vi "FGV_PSP - IPS120 Status.vi"(4 "error in":errorcluster, 6 "Function":enum16{"write", "read"}(ring), 7 "Status":T1) -> (0 "error out":errorcluster, 3 "status":T1)   [LabVIEW 2016, in "IPS-120.lvlib" / "IPS-120-API.lvlib"]
uses:
  IPS-120-API.lvlib
  Typedefs/Status - Cluster.ctl
panel:
  # "Disabled calls to PSP 4/13/2018"
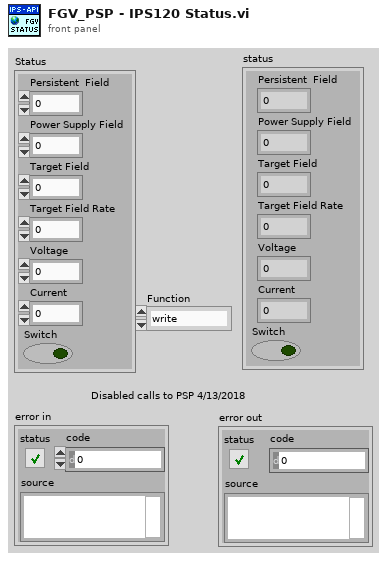
[diagram p1: front panel]
types:
  T1 = typedef "IPS-120.lvlib/IPS-120-API.lvlib/Status - Cluster.ctl" = cluster{"Persistent  Field":dbl, "Power Supply Field":dbl, "Target Field":dbl, "Target Field Rate":dbl, "Voltage":dbl, "Current":dbl, "Switch":bool}
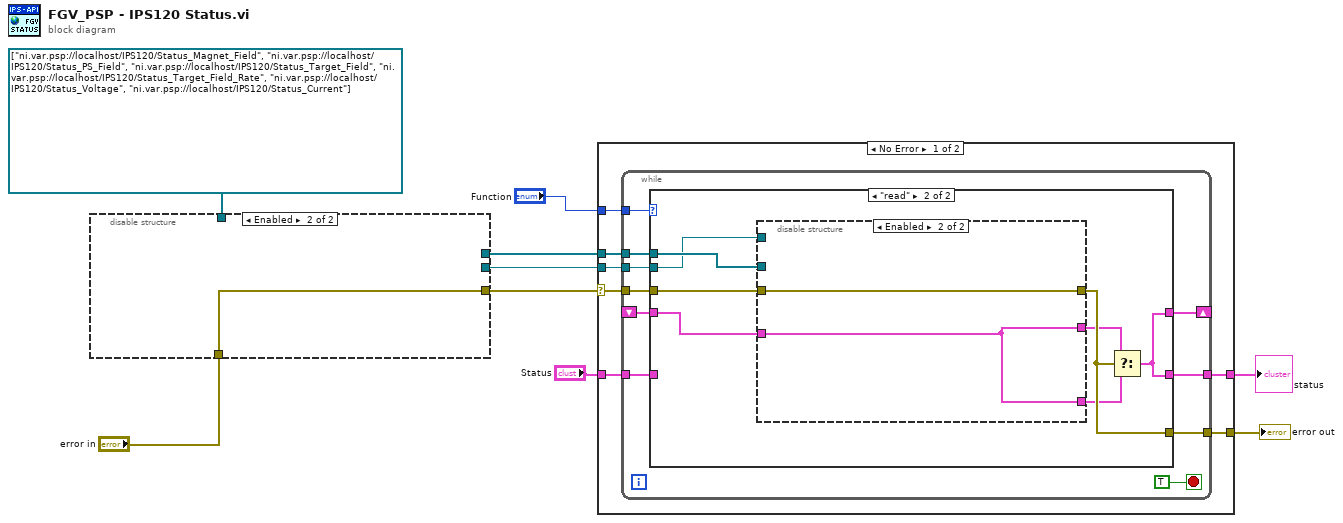
[diagram p0: block diagram]
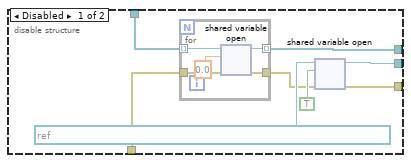
[diagram p2: hidden frame]
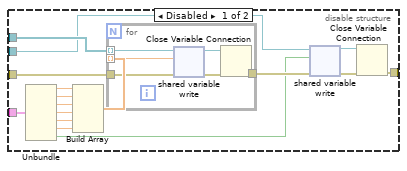
[diagram p4: hidden frame]
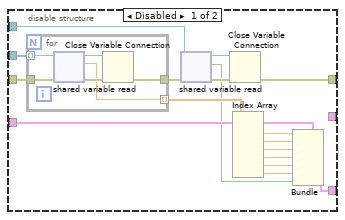
[diagram p5: hidden frame]
diagram:
  n1 = disable-structure shown="Enabled" {
    disable-tunnel: refnum<k21>[] ["ni.var.psp://localhost/IPS120/Status_Magnet_Field", "ni.var.psp://localhost/IPS120/Status_PS_Field", "ni.var.psp://localhost/IPS120/Status_Target_Field", "ni.var.psp://localhost/IPS120/Status_Target_Field_Rate", "ni.var.psp://localhost/IPS120/Status_Voltage", "ni.var.psp://localhost/IPS120/Status_Current"] -> [w16 _]
    disable-tunnel: "error in" -> [w13 w23]
    disable-tunnel: [w12 _] -> w3
    disable-tunnel: [w11 _] -> w2
    disable-tunnel: [w10 w23] -> w1
    frame Disabled {
      n2 = for {
        tunnel: w16 -> [w22] mode=indexing
        tunnel: [w20] -> w12 mode=indexing
        tunnel: [w19] -> w14
        tunnel: w13 -> [w18]
        n3 = shared-variable-open(w22, w18, 0.0) -> (w20:refnum<k21>, w19:errorcluster)  [unwired: 1 in]
      }
      n4 = shared-variable-open(refnum<k21> "ni.var.psp://localhost/IPS120/Status_Switch" ("shared variable refnum in"), w14, TRUE) -> (w11:refnum<k21>, w10:errorcluster)  [unwired: 1 in]
    }
    frame Enabled {
    }
  }
  n5 = case shown="No Error" w1 {
    selector: w1 -> [w30 w103]
    tunnel: [w29 w103] -> w9
    tunnel: "Status" -> [w28 w102]
    tunnel: [w27 w102] -> w6
    tunnel: "Function" -> [w26 _]
    tunnel: w3 -> [w25 _]
    tunnel: w2 -> [w24 _]
    frame No Error {
      n6 = while {
        shift-right: [w34] -> _
        shift-left: _ -> [w33]
        tunnel: w30 -> [w39]
        tunnel: [w38] -> w29
        tunnel: w28 -> [w37]
        tunnel: [w36] -> w27
        tunnel: w26 -> [w35]
        tunnel: w25 -> [w32]
        tunnel: w24 -> [w31]
        stop <- TRUE stop-if-true
        n7 = case shown="\"read\"" w35 {
          tunnel: w39 -> [w43 w73]
          tunnel: [w42 w72] -> w38
          tunnel: w37 -> [w45 _]
          tunnel: [w45 w74] -> w36
          tunnel: [w45 w74] -> w34
          tunnel: w33 -> [_ w75]
          tunnel: w32 -> [w44 w76]
          tunnel: w31 -> [w41 w71]
          frame "write", Default {
            n8 = disable-structure shown="Enabled" {
              disable-tunnel: w45 -> [w61 _]
              disable-tunnel: w44 -> [w54 _]
              disable-tunnel: w43 -> [w49 w68]
              disable-tunnel: [w48 w68] -> w42
              disable-tunnel: w41 -> [w47 _]
              frame Disabled {
                n9 = Unbundle(w61) -> ("Persistent  Field"=w60:dbl, "Power Supply Field"=w55:dbl, "Target Field"=w56:dbl, "Target Field Rate"=w57:dbl, "Voltage"=w58:dbl, "Current"=w59:dbl, "Switch"=w50:bool)
                n10 = Build Array(w60, w55, w56, w57, w58, w59) -> (w53:dbl[])
                n11 = for {
                  tunnel: w49 -> [w67]
                  tunnel: w54 -> [w64] mode=indexing
                  tunnel: w53 -> [w63] mode=indexing
                  tunnel: [w62] -> w51
                  n12 = shared-variable-write(w64, w67, w63) -> (w65:refnum<k21>, w66:errorcluster)
                  n13 = Close Variable Connection(8:w66, 11:w65) -> (0:w62:errorcluster)
                }
                n14 = shared-variable-write(w47, w51, w50) -> (w46:refnum<k21>, w52:errorcluster)
                n15 = Close Variable Connection(8:w52, 11:w46) -> (0:w48:errorcluster)
              }
              frame Enabled {
              }
            }
          }
          frame "read" {
            n16 = disable-structure shown="Enabled" {
              disable-tunnel: w76 -> [w93 _]
              disable-tunnel: w75 -> [w83 w101]
              disable-tunnel: w73 -> [w81 w100]
              disable-tunnel: [w80 w100] -> w72
              disable-tunnel: w71 -> [w79 _]
              disable-tunnel: [w77 w101] -> w70
              disable-tunnel: [_ w101] -> w69
              frame Disabled {
                n17 = for {
                  tunnel: w93 -> [w99] mode=indexing
                  tunnel: [w95] -> w82 mode=indexing
                  tunnel: [w96] -> w85
                  tunnel: w81 -> [w94]
                  n18 = shared-variable-read(w99, w94) -> (w98:refnum<k21>, w97:errorcluster, w95:dbl)  [unwired: 1 out]
                  n19 = Close Variable Connection(8:w97, 11:w98) -> (0:w96:errorcluster)
                }
                n20 = shared-variable-read(w79, w85) -> (w86:refnum<k21>, w84:errorcluster, w78:bool)  [unwired: 1 out]
                n21 = Close Variable Connection(8:w84, 11:w86) -> (0:w80:errorcluster)
                n22 = Index Array(array=w82) -> (element #1=w92:dbl, element #2=w87:dbl, element #3=w88:dbl, element #4=w89:dbl, element #5=w90:dbl, element #6=w91:dbl)  [unwired: 6 in]
                n23 = Bundle(cluster=w83, "Persistent  Field"=w92, "Power Supply Field"=w87, "Target Field"=w88, "Target Field Rate"=w89, "Voltage"=w90, "Current"=w91, "Switch"=w78) -> (w77:T1)
              }
              frame Enabled {
              }
            }
            n24 = Select(t=w69, s=w72, f=w70) -> (s? t:f=w74:T1)
          }
        }
      }
    }
    frame Error {
    }
  }
  "error out" <- w9
  "status" <- w6
